vi "Autonomous Independent.vi"() -> ()   [LabVIEW 2017]
doc: "This VI is called when autonomous begins, and will automatically be terminated when autonomous ends. You can carry out timed or sensor driven robot movement independently without needing to return to the caller."
uses:
  <vilib>/Rock Robotics/WPI/Utilities/WPI_GetSetVariantRefNum.vi
  <vilib>/Rock Robotics/Network Tables/NT Read String.vi
  <vilib>/Rock Robotics/WPI/RobotDrive/WPI_RobotDriveArcadeDrive_Standard(NoSaturation).vi
  <vilib>/Rock Robotics/Network Tables/NT Write Numeric Array.vi
panel:
  out "Current Movement, for debugging":T1 {"Y Joystick Value" scale=1.0..-1.0; "X Joystick Value" scale=-1.0..1.0}
  in  "Array of robot movements":T2(array[cluster])=[{"X Joystick Value"=0.39393939393939403, "Y Joystick Value"=0.0, "Delay (sec)"=1.0, "Movement Name"="turn"}, {"X Joystick Value"=-0.3737373737373737, "Y Joystick Value"=0.0, "Delay (sec)"=1.0, "Movement Name"="turn back"}] {"Y Joystick Value" scale=1.0..-1.0; "X Joystick Value" scale=-1.0..1.0}
  # "Be sure to right-click and choose Data Operations>>Make Current Value default if you want to save the array values with the VI"
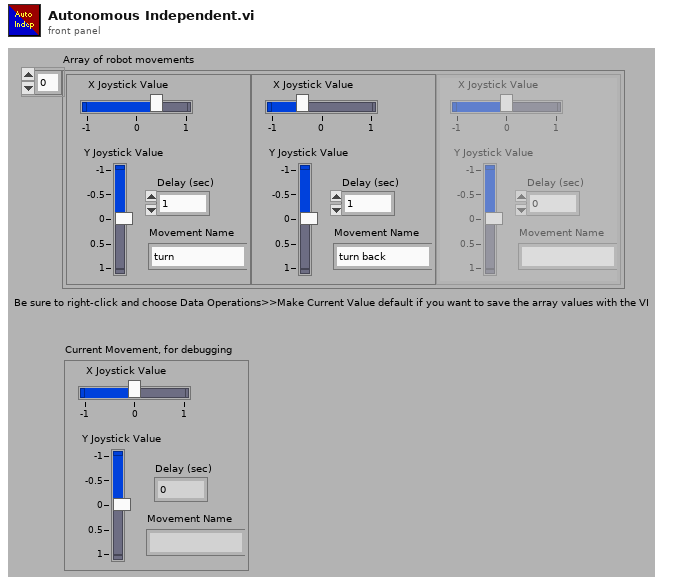
[diagram p1: front panel]
types:
  T1 = cluster{"X Joystick Value":dbl, "Y Joystick Value":dbl, "Delay (sec)":dbl, "Movement Name":string}
  T2 = cluster{"X Joystick Value":dbl, "Y Joystick Value":dbl, "Delay (sec)":dbl, "Movement Name":string}[]
  T3 = typedef "WPI_JoystickDevRef.ctl" = cluster{"Device":T4}
  T4 = typedef "WPI_JoystickDeviceEnum.ctl" = enum16{"USB 0", "USB 1", "USB 2", "USB 3", "USB 4", "USB 5"}
  T5 = typedef "WPI_RobotDriveDevRef.ctl" = cluster{"DevStatus":errorcluster, "Motors[]":T6[], "Square Inputs":bool, "Max Output":dbl}
  T6 = typedef "WPI_MotorControlDeviceRef.ctl" = cluster{"DeviceStatus":errorcluster, "Type":T7, "PWM":cluster{"PWM Channel":T8, "DeadBand":T9}, "CAN":cluster{"Device Number":u8, "SetOutput VI Ref":variant, "GetOutput VI Ref":variant, "Enable VI Ref":variant, "Disable VI Ref":variant, "Data":variant}, "Invert":bool, "DIO PWM":cluster{"PWM \"Enable\" Channel":T8, "DIOChannel":T10, "PWM Rate":dbl}}
  T7 = typedef "WPI_MotorControlType.ctl" = enum16{"PWM", "CAN", "DIO PWM"}
  T8 = typedef "FPGA_DIOPWMChannel.ctl" = enum8{"PWM 0", "PWM 1", "PWM 2", "PWM 3", "PWM 4", "PWM 5", "PWM 6", "PWM 7", "PWM 8", "PWM 9", "PWM MXP 0", "PWM MXP 1", "PWM MXP 2", "PWM MXP 3", "PWM MXP 4", "PWM MXP 5", "PWM MXP 6", "PWM MXP 7", "PWM MXP 8", "PWM MXP 9", "Invalid"}
  T9 = typedef "WPI_PWMDeadband.ctl" = cluster{"Name":string, "maxPositivePwm":i32, "minPositivePwm":i32, "centerPwm":i32, "maxNegativePwm":i32, "minNegativePwm":i32, "angularRange":u16}
  T10 = typedef "FPGA_DIOChannel.ctl" = enum8{"DIO 0", "DIO 1", "DIO 2", "DIO 3", "DIO 4", "DIO 5", "DIO 6", "DIO 7", "DIO 8", "DIO 9", "DIO MXP 0", "DIO MXP 1", "DIO MXP 2", "DIO MXP 3", "DIO MXP 4", "DIO MXP 5", "DIO MXP 6", "DIO MXP 7", "DIO MXP 8", "DIO MXP 9", "DIO MXP 10", "DIO MXP 11", "DIO MXP 12", "DIO MXP 13", "DIO MXP 14", "DIO MXP 15", "SPI Port CS1", "SPI Port CS2", "SPI Port CS3", "SPI Port MISO", "SPI Port MOSI", "Invalid"}
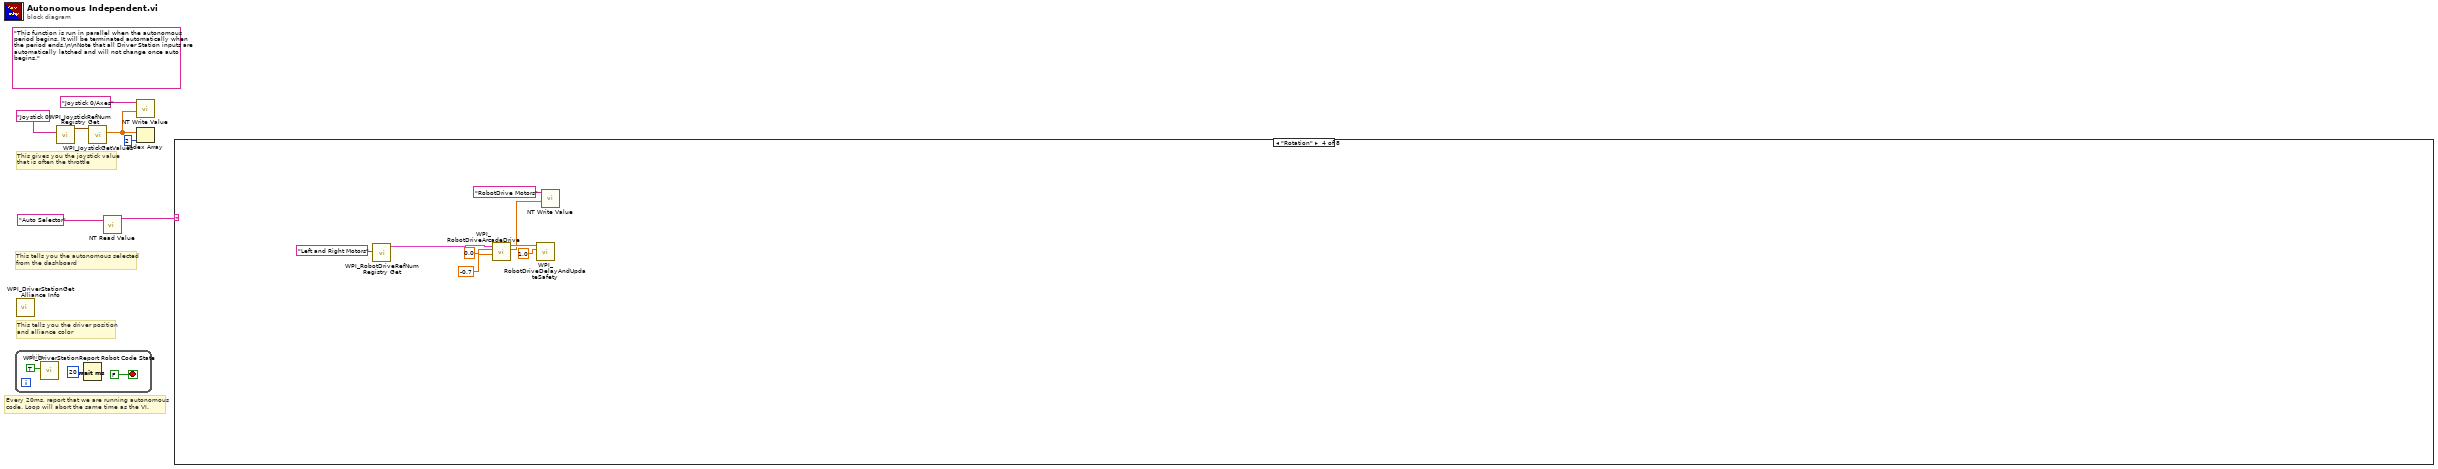
[diagram p0: block diagram]
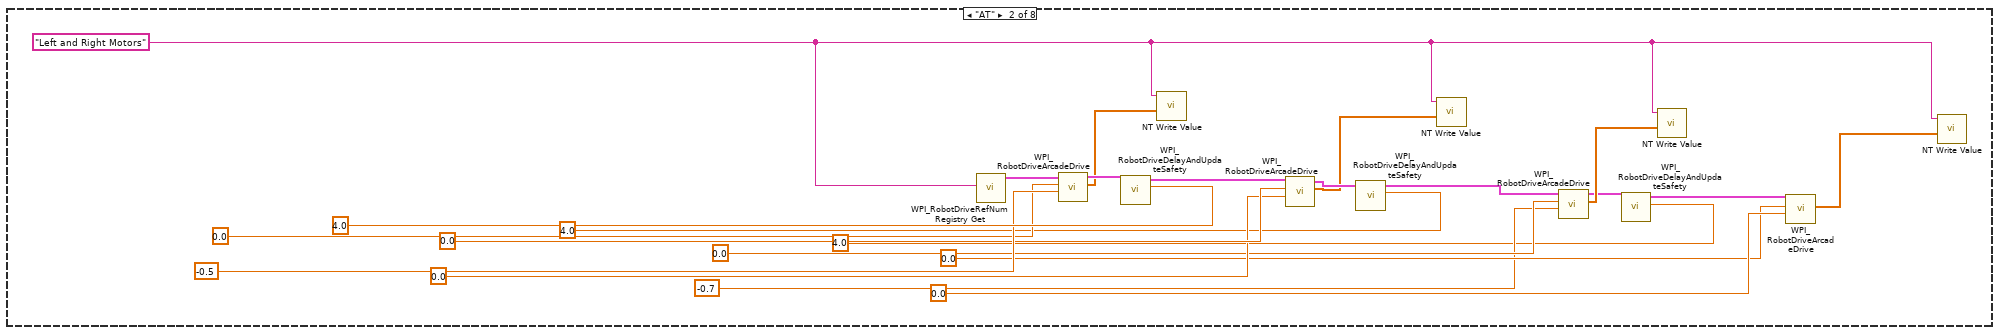
[diagram p3: hidden frame]
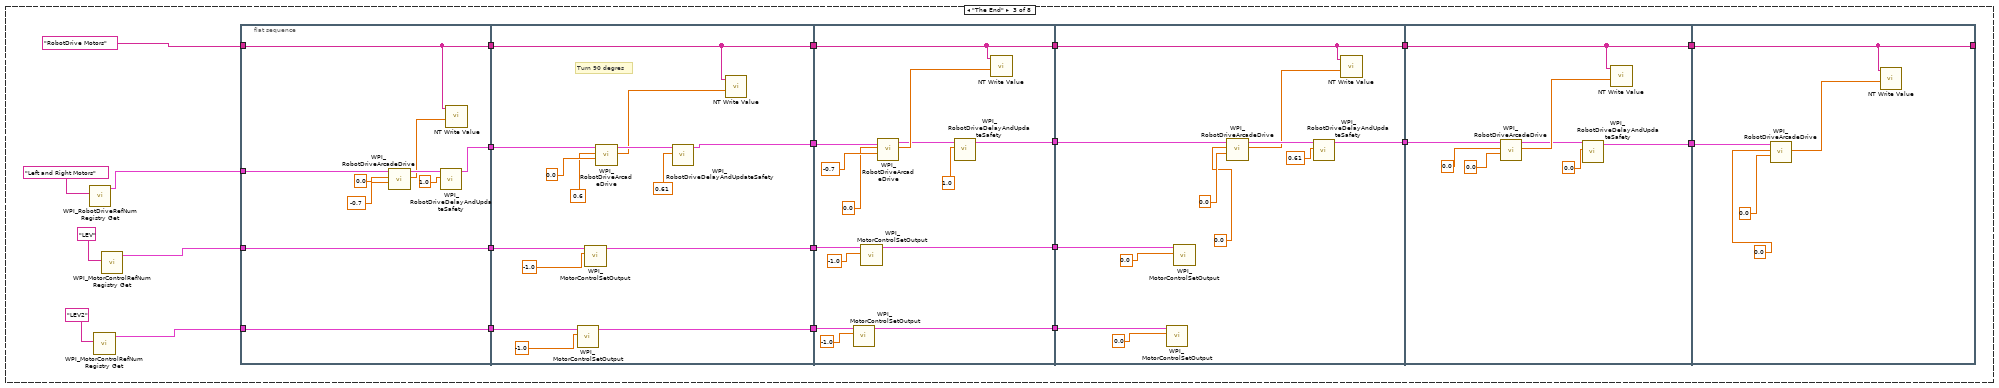
[diagram p4: hidden frame]
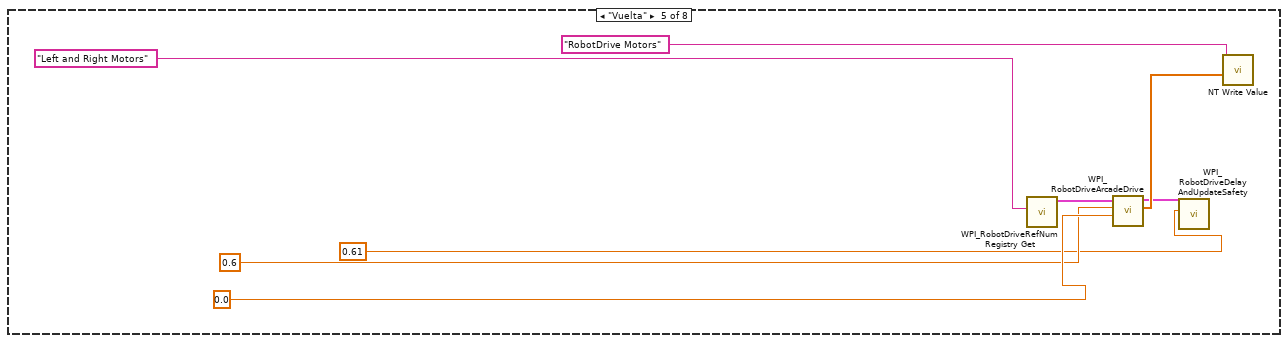
[diagram p5: hidden frame]
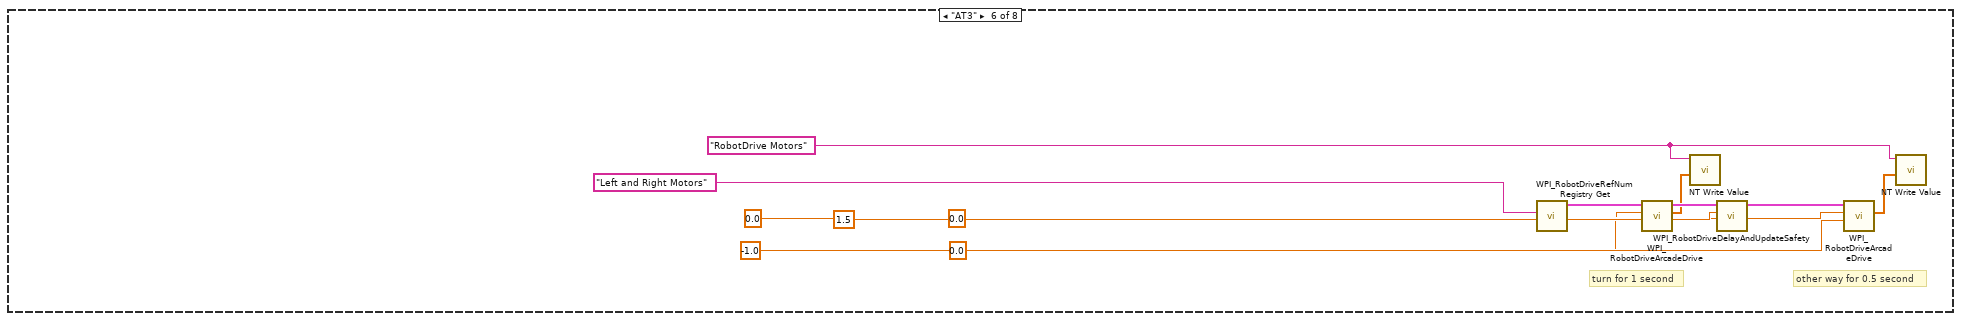
[diagram p6: hidden frame]
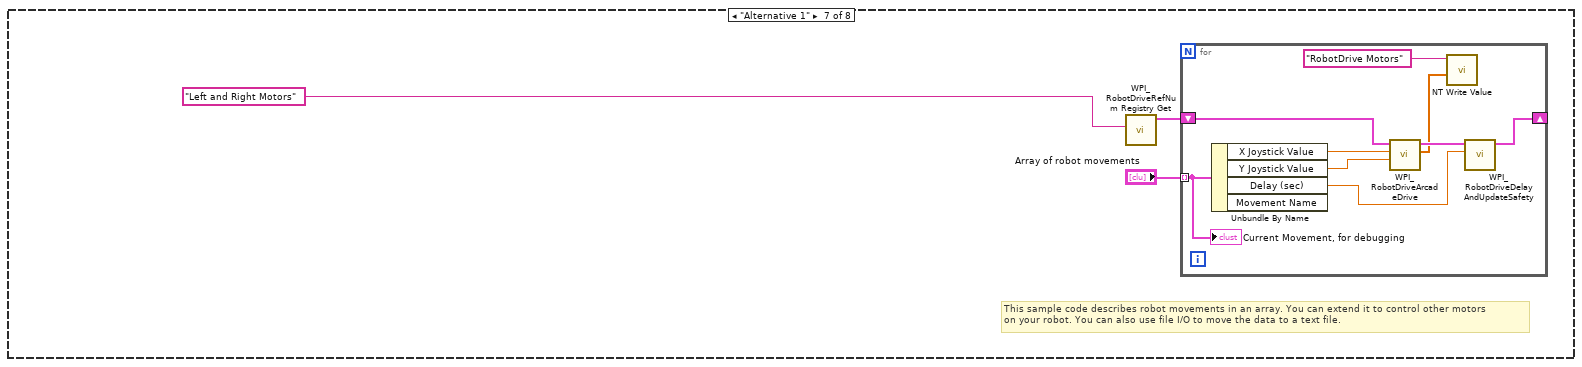
[diagram p7: hidden frame]
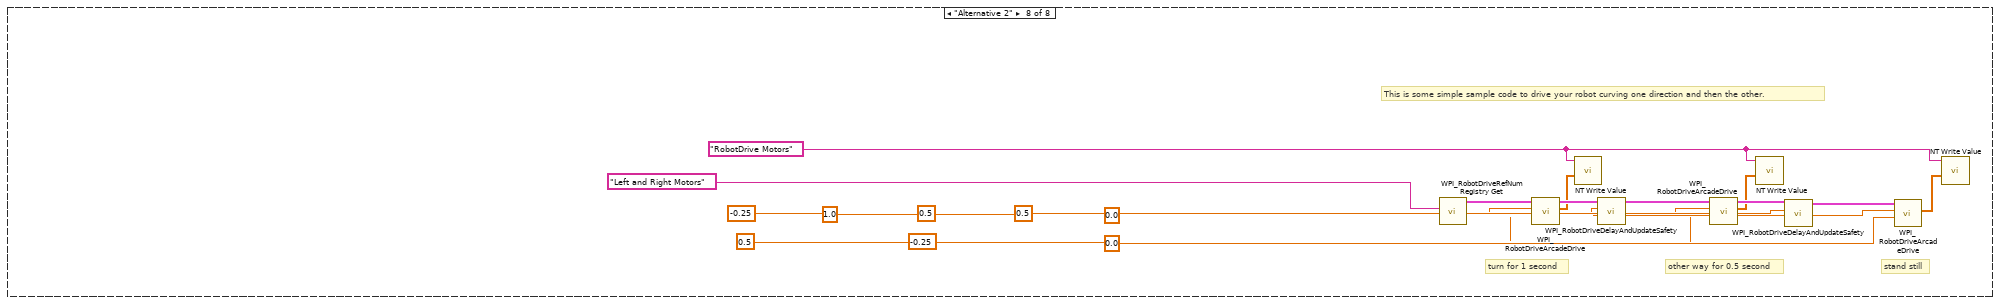
[diagram p8: hidden frame]
diagram:
  (unwired) "This function is run in parallel when the autonomous period begins. It will be terminated automatically when the period ends.\n\nNote that all Driver Station inputs are automatically latched and will not change once auto begins."
  # "This tells you the autonomous selected\nfrom the dashboard"
  # "Every 20ms, report that we are running autonomous\ncode. Loop will abort the same time as the VI."
  # "This gives you the joystick value\nthat is often the throttle"
  # "This tells you the driver position\nand alliance color"
  n1 = while {
    stop <- FALSE stop-if-true
    n2 = call <vilib>:"WPI_DriverStationReport Robot Code State.vi"("Autonomous"=TRUE) -> ()  [unwired: 10 in, 1 out]
    n3 = Wait (ms)(milliseconds to wait=u32 20) -> ()  [unwired: 1 out]
  }
  n4 = call <vilib>:"WPI_DriverStationGet Alliance Info.vi"() -> ()  [unwired: 12 out]
  n5 = call <vilib>:"WPI_JoystickRefNum Registry Get.vi"("refnum name"="Joystick 0") -> ("JoystickDevRef"=w6:T3)  [unwired: 1 in, 9 out]
  n6 = call <vilib>:"WPI_JoystickGetValues.vi"("JoystickDevRef"=w6) -> ("Axes"=w2:dbl[])  [unwired: 6 in, 4 out]
  n7 = call-poly <vilib>:"NT Read Value.vi"("Name"="Auto Selector") -> ("String"=w3:string)  [unwired: 9 in, 1 out]
  n8 = call-poly <vilib>:"NT Write Value.vi"("Numeric Array"=w2, "Name"="Joystick 0/Axes") -> ()  [unwired: 9 in, 1 out]
  n9 = Index Array(array=w2, index=2) -> ()  [unwired: 1 out]
  n10 = case shown="\"Rotation\"" w3 {
    frame Default {
      # "You can put your main auto here, or you can right-click on the case and make any\nother frame be the default case."
      # "This is the frame that will execute if no selection is made, or if it is not recognized"
    }
    frame "AT" {
      w12 = "Left and Right Motors" ("refnum name")
      n11 = call <vilib>:"WPI_RobotDriveRefNum Registry Get.vi"("refnum name"=w12) -> ("RobotDriveDevRef"=w30:T5)  [unwired: 9 in, 1 out]
      n12 = call-poly <vilib>:"WPI_RobotDriveArcadeDrive.vi"("Y axis value"=-0.5, "X axis value"=0.0, "RobotDriveDevRef"=w30) -> ("Motor Values"=w28:dbl[], "RobotDriveDevRef"=w29:T5)  [unwired: 6 in, 1 out]
      n13 = call <vilib>:"WPI_RobotDriveDelayAndUpdateSafety.vi"("Delay (s)"=4.0, "RobotDriveDevRef"=w29) -> ("RobotDriveDevRef 2"=w23:T5)  [unwired: 8 in, 1 out]
      n14 = call-poly <vilib>:"NT Write Value.vi"("Numeric Array"=w28, "Name"=w12) -> ()  [unwired: 9 in, 1 out]
      n15 = call-poly <vilib>:"WPI_RobotDriveArcadeDrive.vi"("Y axis value"=0.0, "X axis value"=0.0, "RobotDriveDevRef"=w23) -> ("Motor Values"=w22:dbl[], "RobotDriveDevRef"=w27:T5)  [unwired: 6 in, 1 out]
      n16 = call <vilib>:"WPI_RobotDriveDelayAndUpdateSafety.vi"("Delay (s)"=4.0, "RobotDriveDevRef"=w27) -> ("RobotDriveDevRef 2"=w11:T5)  [unwired: 8 in, 1 out]
      n17 = call-poly <vilib>:"NT Write Value.vi"("Numeric Array"=w22, "Name"=w12) -> ()  [unwired: 9 in, 1 out]
      n18 = call-poly <vilib>:"WPI_RobotDriveArcadeDrive.vi"("Y axis value"=-0.7, "X axis value"=0.0, "RobotDriveDevRef"=w11) -> ("Motor Values"=w17:dbl[], "RobotDriveDevRef"=w16:T5)  [unwired: 6 in, 1 out]
      n19 = call <vilib>:"WPI_RobotDriveDelayAndUpdateSafety.vi"("Delay (s)"=4.0, "RobotDriveDevRef"=w16) -> ("RobotDriveDevRef 2"=w20:T5)  [unwired: 8 in, 1 out]
      n20 = call-poly <vilib>:"NT Write Value.vi"("Numeric Array"=w17, "Name"=w12) -> ()  [unwired: 9 in, 1 out]
      n21 = call-poly <vilib>:"WPI_RobotDriveArcadeDrive.vi"("Y axis value"=0.0, "X axis value"=0.0, "RobotDriveDevRef"=w20) -> ("Motor Values"=w21:dbl[])  [unwired: 6 in, 2 out]
      n22 = call-poly <vilib>:"NT Write Value.vi"("Numeric Array"=w21, "Name"=w12) -> ()  [unwired: 9 in, 1 out]
    }
    frame "The End" {
      n23 = call <vilib>:"WPI_RobotDriveRefNum Registry Get.vi"("refnum name"="Left and Right Motors") -> ("RobotDriveDevRef"=w52:T5)  [unwired: 1 in, 9 out]
      n24 = call <vilib>:"WPI_MotorControlRefNum Registry Get.vi"("refnum name"="LEV2") -> ("MotorControlDevRef"=w35:T6)  [unwired: 9 in, 1 out]
      n25 = call <vilib>:"WPI_MotorControlRefNum Registry Get.vi"("refnum name"="LEV") -> ("MotorControlDevRef"=w44:T6)  [unwired: 9 in, 1 out]
      n26 = flat-sequence {
        tunnel: [w57] -> w53
        tunnel: w52 -> [w61]
        tunnel: "RobotDrive Motors" ("Name") -> [w59]
        tunnel: [w59] -> w50
        tunnel: w44 -> [w60]
        tunnel: [w60] -> w45
        tunnel: [w58] -> w36
        tunnel: w35 -> [w58]
        tunnel: [w75] -> w54
        tunnel: w53 -> [w74]
        tunnel: w50 -> [w72]
        tunnel: [w72] -> w49
        tunnel: w45 -> [w73]
        tunnel: [w71] -> w39
        tunnel: [w70] -> w37
        tunnel: w36 -> [w69]
        tunnel: w54 -> [w88]
        tunnel: w49 -> [w85]
        tunnel: [w94] -> w48
        tunnel: [w86] -> w47
        tunnel: [w85] -> w46
        tunnel: w39 -> [w84]
        tunnel: [w81] -> w38
        tunnel: w37 -> [w83]
        tunnel: w48 -> [w102]
        tunnel: w47 -> [w99]
        tunnel: w46 -> [w97]
        tunnel: [w97] -> w43
        tunnel: [w98] -> w42
        tunnel: w38 -> [w96]
        tunnel: w43 -> [w107]
        tunnel: w42 -> [w109]
        tunnel: [w107] -> w41
        tunnel: [w108] -> w40
        tunnel: [w115] -> _
        tunnel: w41 -> [w115]
        tunnel: w40 -> [w116]
        frame #0 {
          n27 = call-poly <vilib>:"WPI_RobotDriveArcadeDrive.vi"("Y axis value"=-0.7 ("X axis value"), "X axis value"=0.0, "RobotDriveDevRef"=w61) -> ("Motor Values"=w65:dbl[], "RobotDriveDevRef"=w66:T5)  [unwired: 1 in, 6 out]
          n28 = call <vilib>:"WPI_RobotDriveDelayAndUpdateSafety.vi"("Delay (s)"=1.0, "RobotDriveDevRef"=w66) -> ("RobotDriveDevRef 2"=w57:T5)  [unwired: 8 in, 1 out]
          n29 = call-poly <vilib>:"NT Write Value.vi"("Numeric Array"=w65, "Name"=w59) -> ()  [unwired: 9 in, 1 out]
        }
        frame #1 {
          # "Turn 90 degres"
          n30 = call <vilib>:"WPI_MotorControlSetOutput.vi"("Output"=-1.0 ("X axis value"), "MotorControlDevRef"=w69) -> ("MotorControlDevRef"=w70:T6)  [unwired: 7 in, 2 out]
          n31 = call <vilib>:"WPI_MotorControlSetOutput.vi"("Output"=-1.0 ("X axis value"), "MotorControlDevRef"=w73) -> ("MotorControlDevRef"=w71:T6)  [unwired: 7 in, 2 out]
          n32 = call-poly <vilib>:"WPI_RobotDriveArcadeDrive.vi"("Y axis value"=0.0, "X axis value"=0.6, "RobotDriveDevRef"=w74) -> ("Motor Values"=w79:dbl[], "RobotDriveDevRef"=w80:T5)  [unwired: 6 in, 1 out]
          n33 = call <vilib>:"WPI_RobotDriveDelayAndUpdateSafety.vi"("Delay (s)"=0.61, "RobotDriveDevRef"=w80) -> ("RobotDriveDevRef 2"=w75:T5)  [unwired: 8 in, 1 out]
          n34 = call-poly <vilib>:"NT Write Value.vi"("Numeric Array"=w79, "Name"=w72) -> ()  [unwired: 9 in, 1 out]
        }
        frame #2 {
          n35 = call <vilib>:"WPI_MotorControlSetOutput.vi"("Output"=-1.0 ("X axis value"), "MotorControlDevRef"=w83) -> ("MotorControlDevRef"=w81:T6)  [unwired: 7 in, 2 out]
          n36 = call <vilib>:"WPI_MotorControlSetOutput.vi"("Output"=-1.0 ("X axis value"), "MotorControlDevRef"=w84) -> ("MotorControlDevRef"=w94:T6)  [unwired: 7 in, 2 out]
          n37 = call-poly <vilib>:"WPI_RobotDriveArcadeDrive.vi"("Y axis value"=-0.7, "X axis value"=0.0, "RobotDriveDevRef"=w88) -> ("Motor Values"=w93:dbl[], "RobotDriveDevRef"=w92:T5)  [unwired: 6 in, 1 out]
          n38 = call <vilib>:"WPI_RobotDriveDelayAndUpdateSafety.vi"("Delay (s)"=1.0, "RobotDriveDevRef"=w92) -> ("RobotDriveDevRef 2"=w86:T5)  [unwired: 8 in, 1 out]
          n39 = call-poly <vilib>:"NT Write Value.vi"("Numeric Array"=w93, "Name"=w85) -> ()  [unwired: 9 in, 1 out]
        }
        frame #3 {
          n40 = call <vilib>:"WPI_MotorControlSetOutput.vi"("Output"=0.0 ("LeftSpeed"), "MotorControlDevRef"=w96) -> ()  [unwired: 7 in, 3 out]
          n41 = call <vilib>:"WPI_MotorControlSetOutput.vi"("Output"=0.0 ("LeftSpeed"), "MotorControlDevRef"=w102) -> ()  [unwired: 7 in, 3 out]
          n42 = call-poly <vilib>:"WPI_RobotDriveArcadeDrive.vi"("Y axis value"=0.0, "X axis value"=0.0, "RobotDriveDevRef"=w99) -> ("Motor Values"=w105:dbl[], "RobotDriveDevRef"=w106:T5)  [unwired: 6 in, 1 out]
          n43 = call <vilib>:"WPI_RobotDriveDelayAndUpdateSafety.vi"("Delay (s)"=0.61, "RobotDriveDevRef"=w106) -> ("RobotDriveDevRef 2"=w98:T5)  [unwired: 8 in, 1 out]
          n44 = call-poly <vilib>:"NT Write Value.vi"("Numeric Array"=w105, "Name"=w97) -> ()  [unwired: 9 in, 1 out]
        }
        frame #4 {
          n45 = call-poly <vilib>:"WPI_RobotDriveArcadeDrive.vi"("Y axis value"=0.0, "X axis value"=0.0, "RobotDriveDevRef"=w109) -> ("Motor Values"=w114:dbl[], "RobotDriveDevRef"=w113:T5)  [unwired: 6 in, 1 out]
          n46 = call <vilib>:"WPI_RobotDriveDelayAndUpdateSafety.vi"("Delay (s)"=0.0, "RobotDriveDevRef"=w113) -> ("RobotDriveDevRef 2"=w108:T5)  [unwired: 8 in, 1 out]
          n47 = call-poly <vilib>:"NT Write Value.vi"("Numeric Array"=w114, "Name"=w107) -> ()  [unwired: 9 in, 1 out]
        }
        frame #5 {
          n48 = call-poly <vilib>:"WPI_RobotDriveArcadeDrive.vi"("Y axis value"=0.0, "X axis value"=0.0, "RobotDriveDevRef"=w116) -> ("Motor Values"=w119:dbl[])  [unwired: 6 in, 2 out]
          n49 = call-poly <vilib>:"NT Write Value.vi"("Numeric Array"=w119, "Name"=w115) -> ()  [unwired: 9 in, 1 out]
        }
      }
    }
    frame "Rotation" {
      n50 = call <vilib>:"WPI_RobotDriveRefNum Registry Get.vi"("refnum name"="Left and Right Motors") -> ("RobotDriveDevRef"=w121:T5)  [unwired: 9 in, 1 out]
      n51 = call-poly <vilib>:"WPI_RobotDriveArcadeDrive.vi"("Y axis value"=-0.7 ("X axis value"), "X axis value"=0.0, "RobotDriveDevRef"=w121) -> ("Motor Values"=w126:dbl[], "RobotDriveDevRef"=w127:T5)  [unwired: 1 in, 6 out]
      n52 = call <vilib>:"WPI_RobotDriveDelayAndUpdateSafety.vi"("Delay (s)"=1.0, "RobotDriveDevRef"=w127) -> ()  [unwired: 8 in, 2 out]
      n53 = call-poly <vilib>:"NT Write Value.vi"("Numeric Array"=w126, "Name"="RobotDrive Motors") -> ()  [unwired: 9 in, 1 out]
    }
    frame "Vuelta" {
      n54 = call <vilib>:"WPI_RobotDriveRefNum Registry Get.vi"("refnum name"="Left and Right Motors") -> ("RobotDriveDevRef"=w133:T5)  [unwired: 9 in, 1 out]
      n55 = call-poly <vilib>:"WPI_RobotDriveArcadeDrive.vi"("Y axis value"=0.0, "X axis value"=0.6, "RobotDriveDevRef"=w133) -> ("Motor Values"=w135:dbl[], "RobotDriveDevRef"=w134:T5)  [unwired: 6 in, 1 out]
      n56 = call <vilib>:"WPI_RobotDriveDelayAndUpdateSafety.vi"("Delay (s)"=0.61, "RobotDriveDevRef"=w134) -> ()  [unwired: 8 in, 2 out]
      n57 = call-poly <vilib>:"NT Write Value.vi"("Numeric Array"=w135, "Name"="RobotDrive Motors") -> ()  [unwired: 9 in, 1 out]
    }
    frame "AT3" {
      w142 = "RobotDrive Motors" ("Name")
      # "other way for 0.5 second"
      # "turn for 1 second"
      n58 = call <vilib>:"WPI_RobotDriveRefNum Registry Get.vi"("refnum name"="Left and Right Motors") -> ("RobotDriveDevRef"=w147:T5)  [unwired: 1 in, 9 out]
      n59 = call-poly <vilib>:"WPI_RobotDriveArcadeDrive.vi"("Y axis value"=-1.0 ("X axis value"), "X axis value"=0.0, "RobotDriveDevRef"=w147) -> ("Motor Values"=w143:dbl[], "RobotDriveDevRef"=w145:T5)  [unwired: 1 in, 6 out]
      n60 = call-poly <vilib>:"NT Write Value.vi"("Numeric Array"=w143, "Name"=w142) -> ()  [unwired: 9 in, 1 out]
      n61 = call <vilib>:"WPI_RobotDriveDelayAndUpdateSafety.vi"("Delay (s)"=1.5, "RobotDriveDevRef"=w145) -> ("RobotDriveDevRef 2"=w146:T5)  [unwired: 8 in, 1 out]
      n62 = call-poly <vilib>:"WPI_RobotDriveArcadeDrive.vi"("Y axis value"=0.0 ("X axis value"), "X axis value"=0.0, "RobotDriveDevRef"=w146) -> ("Motor Values"=w144:dbl[])  [unwired: 1 in, 7 out]
      n63 = call-poly <vilib>:"NT Write Value.vi"("Numeric Array"=w144, "Name"=w142) -> ()  [unwired: 9 in, 1 out]
    }
    frame "Alternative 1" {
      # "This sample code describes robot movements in an array. You can extend it to control other motors\non your robot. You can also use file I/O to move the data to a text file."
      n64 = call <vilib>:"WPI_RobotDriveRefNum Registry Get.vi"("refnum name"="Left and Right Motors") -> ("RobotDriveDevRef"=w149:T5)  [unwired: 1 in, 9 out]
      n65 = for {
        shift-right: [w157] -> _
        shift-left: w149 -> [w158]
        tunnel: "Array of robot movements" -> [w153] mode=indexing
        n66 = Unbundle By Name(w153) -> ("X Joystick Value"=w156:dbl, "Y Joystick Value"=w155:dbl, "Delay (sec)"=w154:dbl)  [unwired: 1 out]
        n67 = call-poly <vilib>:"WPI_RobotDriveArcadeDrive.vi"("Y axis value"=w155, "X axis value"=w156, "RobotDriveDevRef"=w158) -> ("Motor Values"=w151:dbl[], "RobotDriveDevRef"=w159:T5)  [unwired: 1 in, 6 out]
        n68 = call-poly <vilib>:"NT Write Value.vi"("Numeric Array"=w151, "Name"="RobotDrive Motors") -> ()  [unwired: 9 in, 1 out]
        n69 = call <vilib>:"WPI_RobotDriveDelayAndUpdateSafety.vi"("Delay (s)"=w154, "RobotDriveDevRef"=w159) -> ("RobotDriveDevRef 2"=w157:T5)  [unwired: 8 in, 1 out]
        "Current Movement, for debugging" <- w153
      }
    }
    frame "Alternative 2" {
      w161 = "RobotDrive Motors" ("Name")
      # "This is some simple sample code to drive your robot curving one direction and then the other."
      # "stand still"
      # "other way for 0.5 second"
      # "turn for 1 second"
      n70 = call <vilib>:"WPI_RobotDriveRefNum Registry Get.vi"("refnum name"="Left and Right Motors") -> ("RobotDriveDevRef"=w177:T5)  [unwired: 1 in, 9 out]
      n71 = call-poly <vilib>:"WPI_RobotDriveArcadeDrive.vi"("Y axis value"=0.5 ("X axis value"), "X axis value"=-0.25, "RobotDriveDevRef"=w177) -> ("Motor Values"=w160:dbl[], "RobotDriveDevRef"=w170:T5)  [unwired: 1 in, 6 out]
      n72 = call-poly <vilib>:"NT Write Value.vi"("Numeric Array"=w160, "Name"=w161) -> ()  [unwired: 9 in, 1 out]
      n73 = call <vilib>:"WPI_RobotDriveDelayAndUpdateSafety.vi"("Delay (s)"=1.0, "RobotDriveDevRef"=w170) -> ("RobotDriveDevRef 2"=w171:T5)  [unwired: 8 in, 1 out]
      n74 = call-poly <vilib>:"WPI_RobotDriveArcadeDrive.vi"("Y axis value"=-0.25 ("X axis value"), "X axis value"=0.5, "RobotDriveDevRef"=w171) -> ("Motor Values"=w162:dbl[], "RobotDriveDevRef"=w172:T5)  [unwired: 1 in, 6 out]
      n75 = call-poly <vilib>:"NT Write Value.vi"("Numeric Array"=w162, "Name"=w161) -> ()  [unwired: 9 in, 1 out]
      n76 = call <vilib>:"WPI_RobotDriveDelayAndUpdateSafety.vi"("Delay (s)"=0.5, "RobotDriveDevRef"=w172) -> ("RobotDriveDevRef 2"=w173:T5)  [unwired: 8 in, 1 out]
      n77 = call-poly <vilib>:"WPI_RobotDriveArcadeDrive.vi"("Y axis value"=0.0 ("X axis value"), "X axis value"=0.0, "RobotDriveDevRef"=w173) -> ("Motor Values"=w163:dbl[])  [unwired: 1 in, 7 out]
      n78 = call-poly <vilib>:"NT Write Value.vi"("Numeric Array"=w163, "Name"=w161) -> ()  [unwired: 9 in, 1 out]
    }
  }
